vi "main_forSimulation.vi"() -> ()   [LabVIEW 2012]
panel:
  in  "stop":bool
  in  "Tank2AqFind":bool
  in  "Tank2AqAngle":dbl
  in  "Tank2":dbl[](array[numeric])=[-1.0, -1.0]
  in  "Tank1AqFind":bool
  in  "Tank1AqAngle":dbl
  in  "Tank1":dbl[](array[numeric])=[1.0, 1.0]
  in  "K":i16
  in  "dir2":dbl
  in  "dir1":dbl
  in  "Ball":dbl[](array[numeric])=[0.0, 0.0]
  # "1. 打开间谍卫星系统"
  # "2. 打开两个机器人的IPcamera"
  # "这里暂时手调"
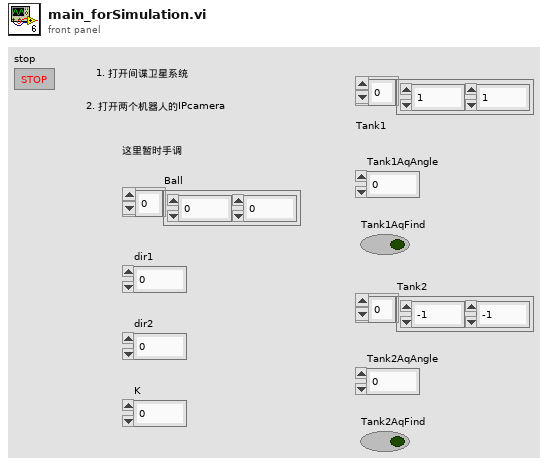
[diagram p1: front panel]
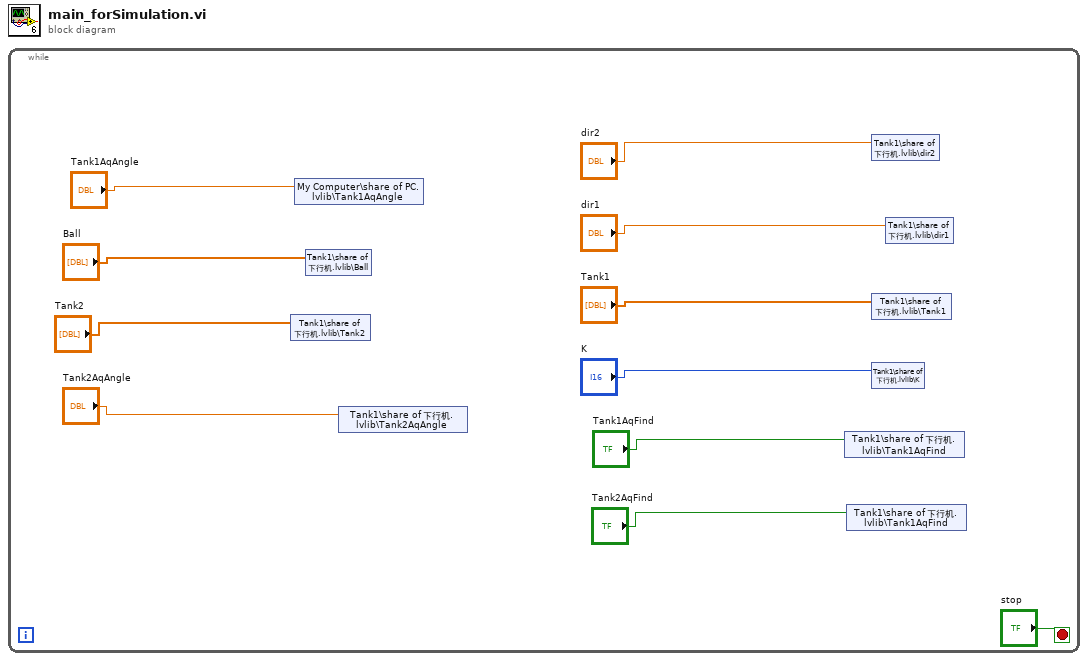
[diagram p0: block diagram]
diagram:
  n1 = while {
    stop <- "stop" stop-if-true
    n2 = shared-variable "Tank1\\share of 下行机.lvlib\\Tank2"("Tank2") -> ()  [unwired: 1 in, 1 out]
    n3 = shared-variable "My Computer\\share of PC.lvlib\\Tank1AqAngle"("Tank1AqAngle") -> ()  [unwired: 1 in, 1 out]
    n4 = shared-variable "Tank1\\share of 下行机.lvlib\\Ball"("Ball") -> ()  [unwired: 1 in, 1 out]
    n5 = shared-variable "Tank1\\share of 下行机.lvlib\\Tank2AqAngle"("Tank2AqAngle") -> ()  [unwired: 1 in, 1 out]
    n6 = shared-variable "Tank1\\share of 下行机.lvlib\\Tank1AqFind"("Tank1AqFind") -> ()  [unwired: 1 in, 1 out]
    n7 = shared-variable "Tank1\\share of 下行机.lvlib\\Tank1AqFind"("Tank2AqFind") -> ()  [unwired: 1 in, 1 out]
    n8 = shared-variable "Tank1\\share of 下行机.lvlib\\dir2"("dir2") -> ()  [unwired: 1 in, 1 out]
    n9 = shared-variable "Tank1\\share of 下行机.lvlib\\Tank1"("Tank1") -> ()  [unwired: 1 in, 1 out]
    n10 = shared-variable "Tank1\\share of 下行机.lvlib\\K"("K") -> ()  [unwired: 1 in, 1 out]
    n11 = shared-variable "Tank1\\share of 下行机.lvlib\\dir1"("dir1") -> ()  [unwired: 1 in, 1 out]
  }
